vi "Partition_Extract.vi"(1 "input cluster":T1={"Core"={"Current VI Reference"=refnum, "Close Panel on Exit?"=FALSE}, "Image Out"=refnum, "State"=0, "Points"={"Top Left"={"X"=0.0, "Y"=0.0}, "Top Right"={"X"=0.0, "Y"=0.0}, "Bottom Left"={"X"=0.0, "Y"=0.0}, "Bottom Right"={"X"=0.0, "Y"=0.0}, "x space 2"=0.0, "y space 2"=0.0, "x_space"=0.0, "y_space"=0.0, "Pixels"=[], "Fixpoint"={"X"=0.0, "Y"=0.0}}, "img_array"=[], "Temps"=[], "Temps_Array"=[], "Scan Area"=0.0, "Fixpoint Area"=0.0, "Config"={"Freezing"={"Cutoff"=2.0, "EndIndex"=2}}, "PCR Size"=0, "ImageCount"=0, "ShowGradient"=FALSE} {"Points"."Bottom Right"."Y" format="%.2f"; "Points"."Bottom Right"."X" format="%.2f"; "Points"."Top Left"."Y" format="%.2f"; "Points"."Top Left"."X" format="%.2f"; "Points"."Top Right"."Y" format="%.2f"; "Points"."Top Right"."X" format="%.2f"; "Points"."Bottom Left"."Y" format="%.2f"; "Points"."Bottom Left"."X" format="%.2f"; "Points"."Fixpoint"."Y" format="%.2f"; "Points"."Fixpoint"."X" format="%.2f"}, 2 "Path":path) -> (0 "PartitionArray":string[](array[string]))   [LabVIEW 2022 SP3]
uses:
  DataCluster_TCAL.ctl
  <vilib>/vision/Image Controls.llb/IMAQ Image.ctl
  TCE_Config.ctl
  <vilib>/Utility/file.llb/Read Delimited Spreadsheet (string).vi
panel:
  out "output array":string[](array[string])
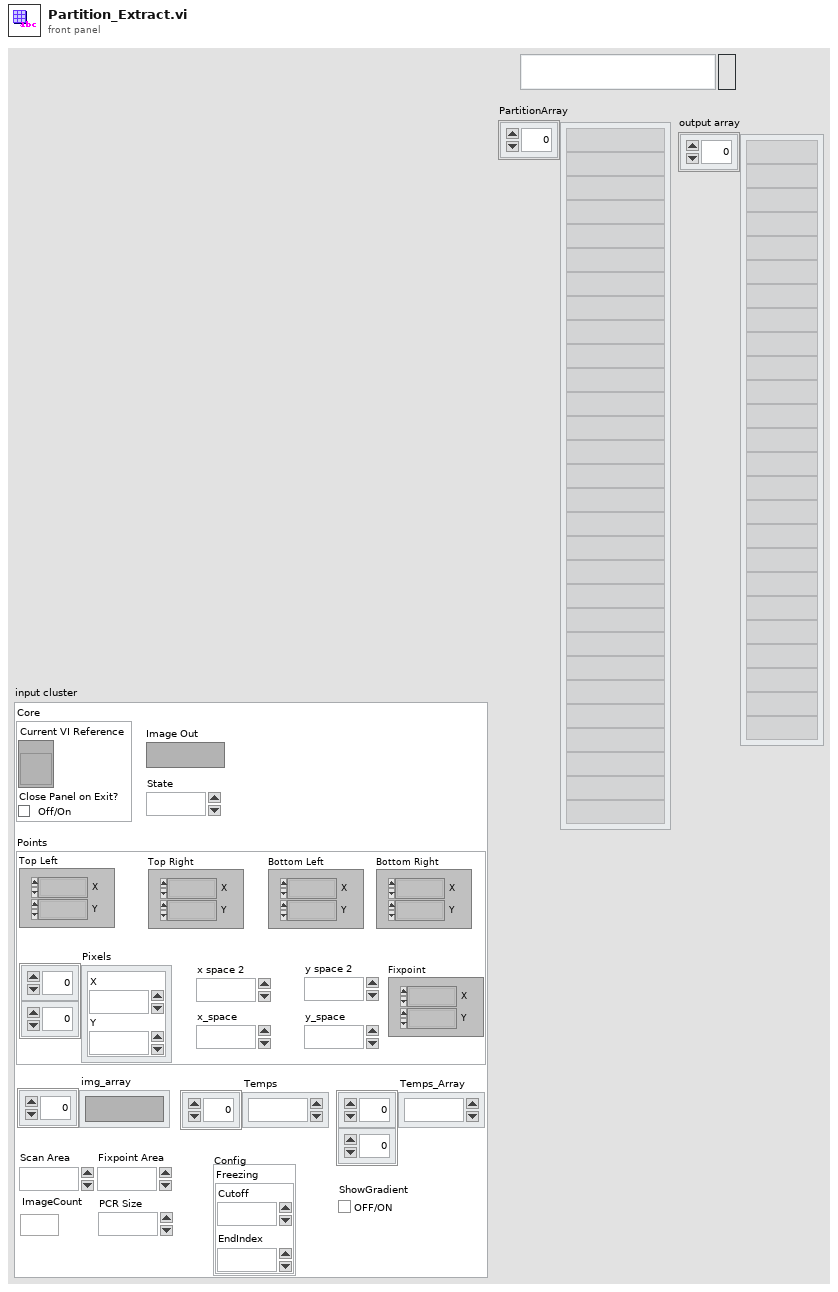
[diagram p1: front panel]
types:
  T1 = typedef "DataCluster_TCAL.ctl" = cluster{"Core":cluster{"Current VI Reference":refnum<vi>, "Close Panel on Exit?":bool}, "Image Out":T2, "State":i32, "Points":cluster{"Top Left":T3, "Top Right":T3, "Bottom Left":T3, "Bottom Right":T3, "x space 2":dbl, "y space 2":sgl, "x_space":sgl, "y_space":sgl, "Pixels":cluster{"X":i32, "Y":i32}[][], "Fixpoint":T3}, "img_array":T2[], "Temps":dbl[], "Temps_Array":dbl[][], "Scan Area":dbl, "Fixpoint Area":dbl, "Config":T4, "PCR Size":u16, "ImageCount":i32, "ShowGradient":bool}
  T2 = typedef "IMAQ Image.ctl" = refnum<image>
  T3 = typedef "IMAQ Point" = cluster{"X":sgl, "Y":sgl}
  T4 = typedef "TCE_Config.ctl" = cluster{"Freezing":cluster{"Cutoff":dbl, "EndIndex":i32}}
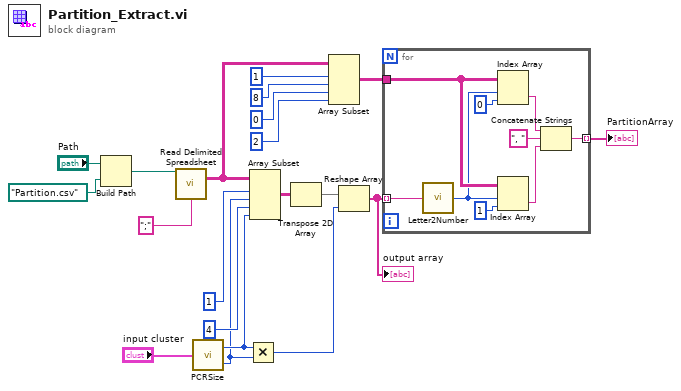
[diagram p0: block diagram]
diagram:
  n1 = Build Path(base path="Path", name or relative path=path "Partition.csv") -> (appended path=w18:path)
  n2 = call-poly <vilib>:"Read Delimited Spreadsheet.vi"("file path (dialog if empty)"=w18, "delimiter (\\t)"=";" ("delimiter (\\t)")) -> ("all rows"=w10:string[][])  [unwired: 8 in, 5 out]
  n3 = call "PCRSize.vi"("input cluster"="input cluster") -> ("Width"=w12:i32, "Height"=w2:i32)
  n4 = Multiply(x=w12, y=w2) -> (x*y=w3:i32)
  n5 = Array Subset(array=w10, index (row)=1 ("index"), length (row)=w2, index (col)=4 ("index"), length (col)=w12) -> (w13:string[][])
  n6 = Transpose 2D Array(2D array=w13) -> (transposed array=w1:string[][])
  n7 = Array Subset(array=w10, index (row)=1 ("index"), length (row)=8 ("length"), index (col)=0 ("index"), length (col)=2 ("length")) -> (w5:string[][])
  n8 = Reshape Array(w1, w3) -> (w11:string[])
  "output array" <- w11
  n9 = for {
    tunnel: w11 -> [w29] mode=indexing
    tunnel: w5 -> [w27]
    tunnel: [w22] -> w4 mode=indexing
    n10 = call "Letter2Number.vi"("Letter"=w29) -> ("Int"=w26:i32)
    n11 = Index Array(array=w27, index (row)=w26, index (col)=0 ("disabled index (col)")) -> (element=w24:string)
    n12 = Index Array(array=w27, index (row)=w26, index (col)=1 ("disabled index (col)")) -> (element=w21:string)
    n13 = Concatenate Strings(w24, ", " ("string"), w21) -> (w22:string)
  }
  "PartitionArray" <- w4
